vi "VisualizeFlags.vi"() -> ()   [LabVIEW 2017, in "Visualization.lvlib" / "VisualizeFlags.lvclass"]
uses:
  VisualizeFlags.lvclass
  Framework/Bus_class/Bus.lvclass
  VisializeBase_class/Typedefs/VisualizeData.ctl
  VisializeBase_class/Typedefs/clVisualizeData.ctl
  Modules/EventPlugins/EventPluginBaseClass/TypeDefs/clEvtReportArray.ctl
  Modules/EventPlugins/EventPluginBaseClass/TypeDefs/clEvtReport.ctl
  Modules/EventPlugins/EventPluginBaseClass/TypeDefs/dblEvtSignalArray.ctl
  Modules/NetworkImpairmentModule/PublicAPI/Arguments/Broadcasts/dblNetworkTime.ctl
  Modules/NetworkImpairmentModule/PublicAPI/Arguments/Broadcasts/dblPktLoss.ctl
  Modules/FlagImpairModule/PublicAPI/Arguments/Broadcasts/ui32FlagImpairmentArray.ctl
  Framework/Bus_class/Broadcast/Typedefs/clDidInit.ctl
  QMH/Typedefs/clFlagImpairArray.ctl
  VisializeBase_class/Requests/clUserEventType.ctl
  <vilib>/event_ctls.llb/usereventprio.ctl
  <vilib>/Utility/miscctls.llb/LVStringsAndValuesArrayTypeDef_U8.ctl
  QMH/Typedefs/clEvtRptArray.ctl
  QMH/Typedefs/clPmuImpairRptArray.ctl
  QMH/Typedefs/clNetImpairmentTime.ctl
  QMH/Typedefs/clNetIPktLoss.ctl
  QMH/Typedefs/clEvtRptSignal.ctl
  <vilib>/Analysis/baseanly.llb/Mean (DBL).vi
  <vilib>/Waveform/DWDTOps.llb/DWDT Boolean Array to Digital.vi
  <vilib>/Utility/error.llb/Error Cluster From Error Code.vi
  <vilib>/ErrorRing/Error Ring.xnode
  VisializeBase_class/VisualizeBase_class.lvclass
  <userlib>/NIST/NISTErrorLib/NISTErrorLib.lvlib
  Framework/Bus_class/Bus_class.lvlib
  Modules/EventModule/EventModule.lvlib
  Modules/PmuImpairModule/PmuImpairModule.lvlib
  Modules/NetworkImpairmentModule/NetworkImpairmentModule.lvlib
  Modules/FlagImpairModule/FlagImpairModule.lvlib
  Modules/EventPlugins/EventPluginBaseClass/EventPluginBaseClass.lvclass
  <vilib>/Analysis/NI_AALBase.lvlib
  VisualizeApp_class/VisualizeAppBase_class.lvclass
panel:
  out "Error Out":errorcluster[](array[cluster])
  in  "Scrollbar":i32(c297)=20
  in  "QueName":string="FlagQue"
  out "Flags":digitalwaveform(graph)={"t0"=timestamp(0 s since 1904-01-01), "dt"=0.016666666666666666, "Y"={"transitions"=[], "data"=array601x32[19232 elements]}}
  in  "Bus Number":u8(ring) items=["", "1"]
  in  "btnStop":bool
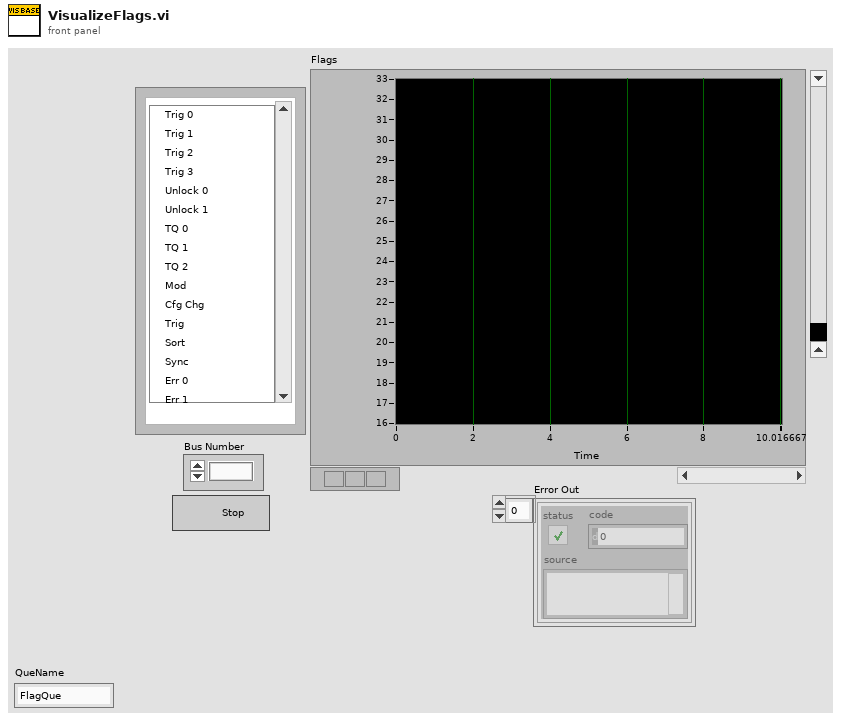
[diagram p1: front panel]
types:
  T1 = typedef "Visualization.lvlib/VisualizeBase_class.lvclass/VisualizeData.ctl" = T2[]
  T2 = typedef "Visualization.lvlib/VisualizeAppBase_class.lvclass/clVisualizeData.ctl" = cluster{"clEvtReportArray":T3, "dblEventSignalArray":T5, "clPmuImpairRptArray":T3, "dblNetworkTime":T6, "dblPktLoss":T7, "FlagImpairArray":T8, "TimeArray":dbl[]}
  T3 = typedef "EventPlugins.lvlib/EventPluginBaseClass.lvclass/clEvtReportArray.ctl" = T4[]
  T4 = typedef "EventPlugins.lvlib/EventPluginBaseClass.lvclass/clEvtReport.ctl" = cluster{"Timestamp":dbl, "Synx":cdb[], "Freq":dbl, "ROCOF":dbl, "ID":i16}
  T5 = typedef "EventPlugins.lvlib/EventPluginBaseClass.lvclass/dblEvtSignalArray.ctl" = dbl[][]
  T6 = typedef "NetworkImpairmentModule.lvlib/dblNetworkTime.ctl" = dbl[]
  T7 = typedef "NetworkImpairmentModule.lvlib/dblPktLoss.ctl" = dbl[]
  T8 = typedef "FlagImpairModule.lvlib/ui32FlagImpairmentArray.ctl" = u32[]
  T9 = typedef "Visualization.lvlib/VisualizeBase_class.lvclass/clRequestEvents.ctl" = cluster{"StopRequest":refnum<user-event>}
  T10 = typedef "Bus_class.lvlib/clBroadcastEvents.ctl" = cluster{"DidInit":refnum<user-event>, "DidStop":refnum<user-event>}
  T11 = typedef "EventModule.lvlib/clBroadcastEvents.ctl" = cluster{"DidInit":refnum<user-event>, "StatusUpdate":refnum<user-event>, "ErrorReport":refnum<user-event>, "DidStop":refnum<user-event>, "ReadEvtConfig":refnum<user-event>, "ReadTimeArray":refnum<user-event>, "ReadEvtParams":refnum<user-event>, "GetEvtReportArray":refnum<user-event>, "ReadPathToPlugin":refnum<user-event>, "GetEvtSignal":refnum<user-event>, "ReadBusNumber":refnum<user-event>}
  T12 = typedef "PmuImpairModule.lvlib/clBroadcastEvents.ctl" = cluster{"DidInit":refnum<user-event>, "StatusUpdate":refnum<user-event>, "ErrorReport":refnum<user-event>, "DidStop":refnum<user-event>, "ImpairConfig":refnum<user-event>, "ImpairParams":refnum<user-event>, "ImpairReports":refnum<user-event>, "PathToPlugin":refnum<user-event>, "BusNumber":refnum<user-event>}
  T13 = typedef "NetworkImpairmentModule.lvlib/clBroadcastEvents.ctl" = cluster{"DidInit":refnum<user-event>, "StatusUpdate":refnum<user-event>, "ErrorReport":refnum<user-event>, "DidStop":refnum<user-event>, "ReadNetImpParams":refnum<user-event>, "ReadLossThreshold":refnum<user-event>, "GetNetworkTime":refnum<user-event>, "GetPktLoss":refnum<user-event>, "ReadPathToPlugin":refnum<user-event>}
  T14 = typedef "FlagImpairModule.lvlib/clBroadcastEvents.ctl" = cluster{"DidInit":refnum<user-event>, "StatusUpdate":refnum<user-event>, "ErrorReport":refnum<user-event>, "DidStop":refnum<user-event>, "ReadFlagImpairConfig":refnum<user-event>, "ReadPluginINIFilePath":refnum<user-event>, "ReadFlagImpairParams":refnum<user-event>, "ReadTimeArray":refnum<user-event>, "GetFlagImpairment":refnum<user-event>}
  T15 = typedef "LVStringsAndValuesArrayTypeDef_U8.ctl" = cluster{"String":string, "Value":u8}[]
  T16 = typedef "Visualization.lvlib/VisualizeBase_class.lvclass/clEvtRptArray.ctl" = cluster{"BusIndex":i32, "clImpairReportArray":T3}
  T17 = typedef "Visualization.lvlib/VisualizeBase_class.lvclass/clPmuImpairRptArray.ctl" = cluster{"BusIndex":i32, "clImpairReportArray":T3}
  T18 = typedef "Visualization.lvlib/VisualizeBase_class.lvclass/clNetImpairmentTime.ctl" = cluster{"BusIndex":i32, "clNetImpairTimeArray":T6}
  T19 = typedef "Visualization.lvlib/VisualizeBase_class.lvclass/clNetIPktLoss.ctl" = cluster{"BusIndex":i32, "clNetPktLoss":T7}
  T20 = typedef "Visualization.lvlib/VisualizeBase_class.lvclass/clFlagImpairArray.ctl" = cluster{"BusIndex":i32, "FlagImpairArray":T8}
  T21 = typedef "Visualization.lvlib/VisualizeBase_class.lvclass/clEvtRptSignal.ctl" = cluster{"BusIndex":i32, "dblEventSignalArray":T5}
  T22 = typedef "Visualization.lvlib/VisualizeBase_class.lvclass/clUserEventType.ctl" = cluster{"BusIndex":i8, "Data":variant}
  T23 = typedef "usereventprio.ctl" = enum32{"high priority", "normal priority"}
  T24 = typedef "Bus_class.lvlib/clDidInit.ctl" = cluster{"Bus":refnum<vi>, "Init?":bool}
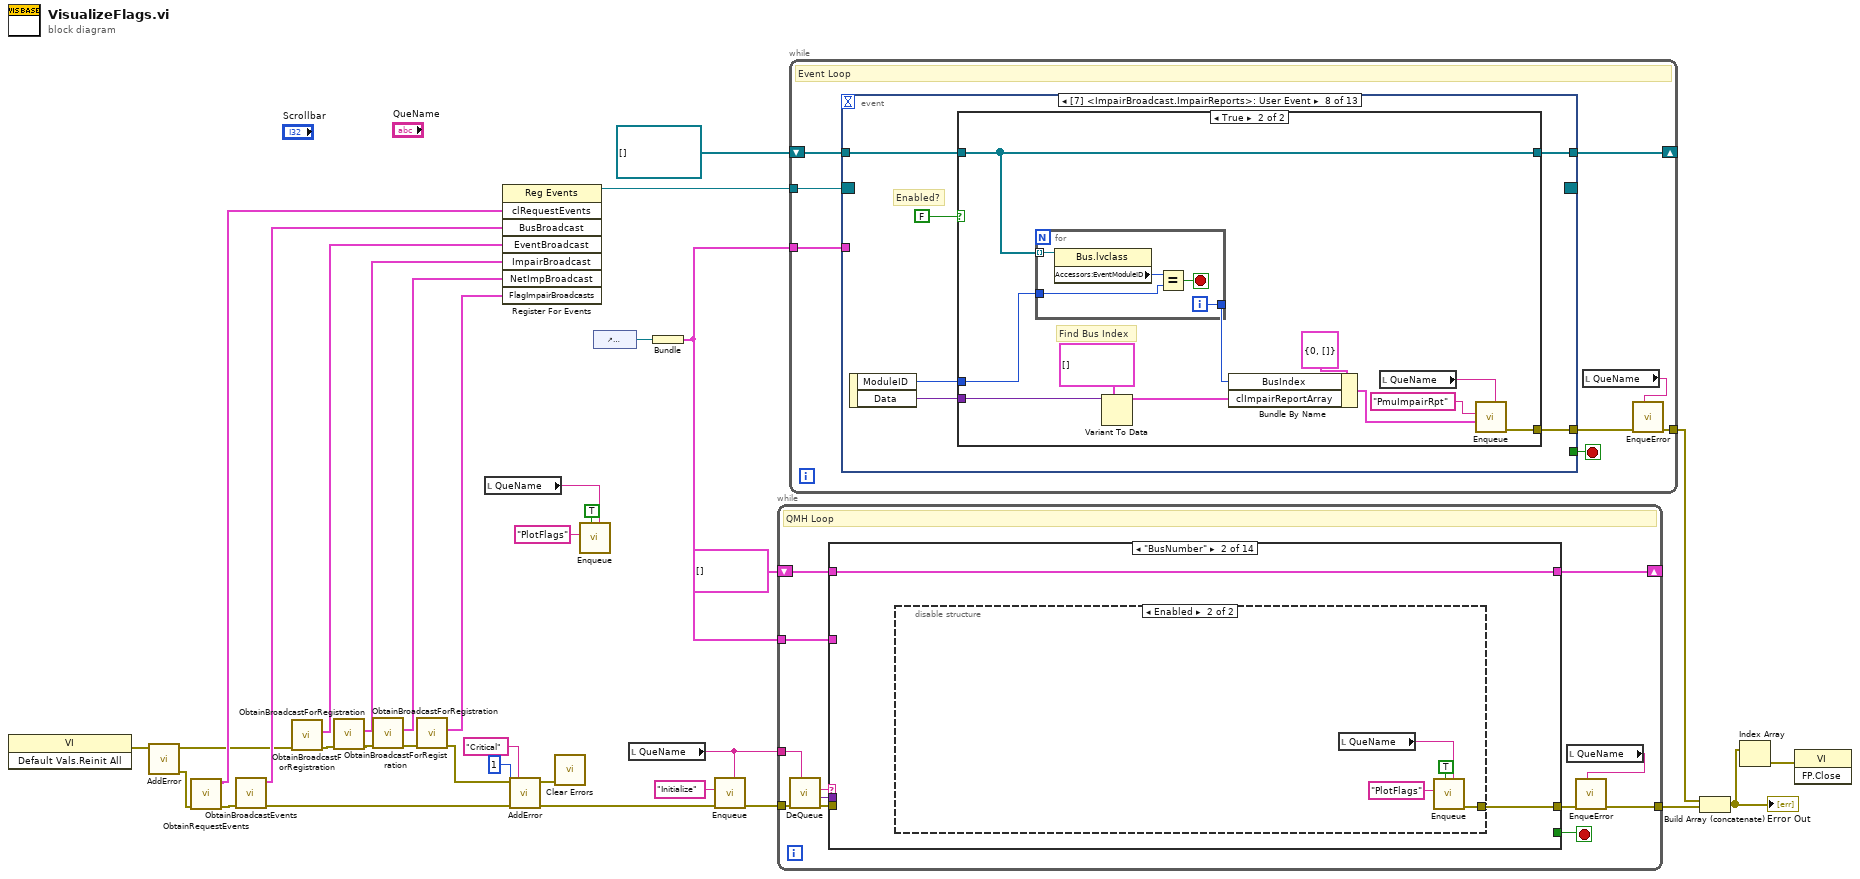
[diagram p0: block diagram]
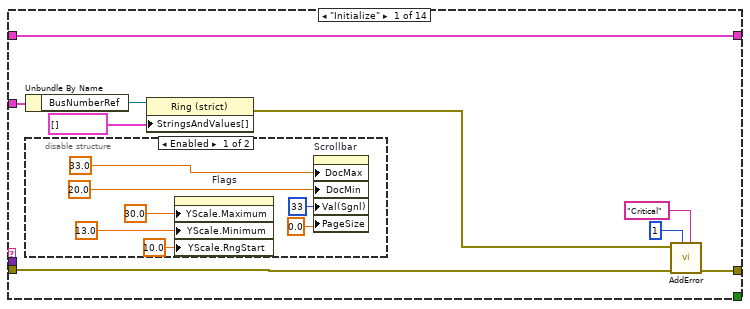
[diagram p2: hidden frame]
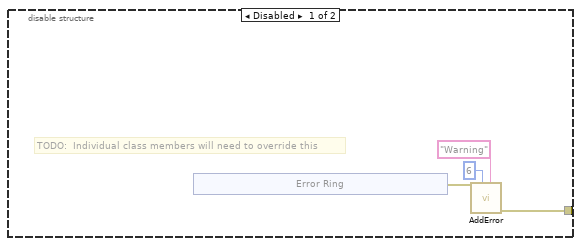
[diagram p4: hidden frame]
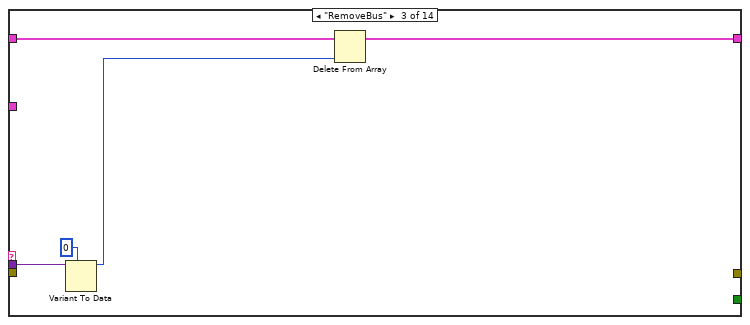
[diagram p5: hidden frame]
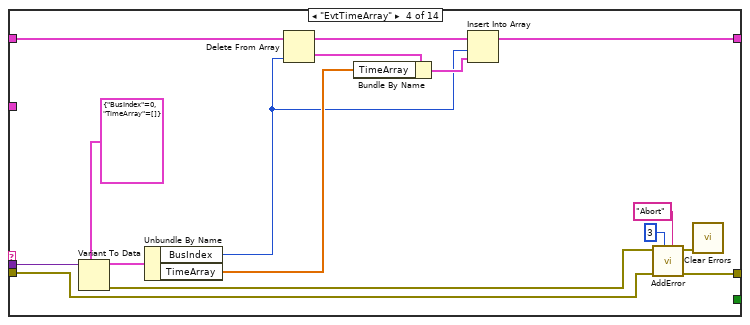
[diagram p6: hidden frame]
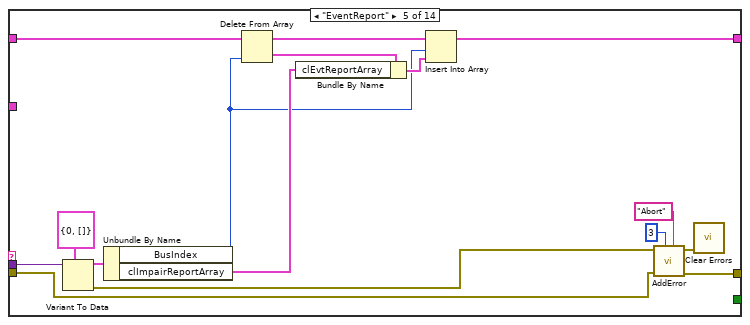
[diagram p7: hidden frame]
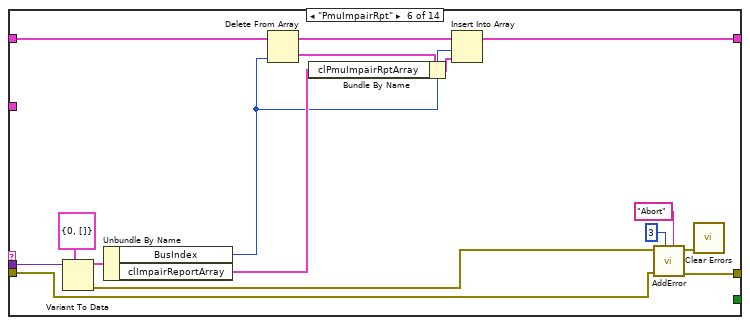
[diagram p8: hidden frame]
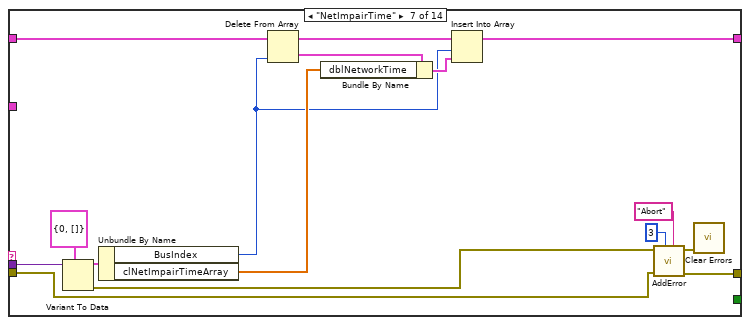
[diagram p9: hidden frame]
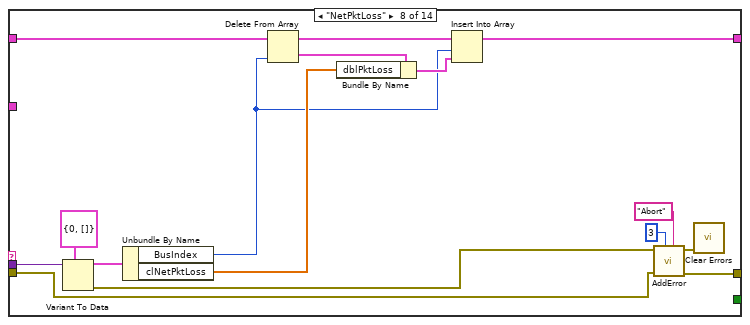
[diagram p10: hidden frame]
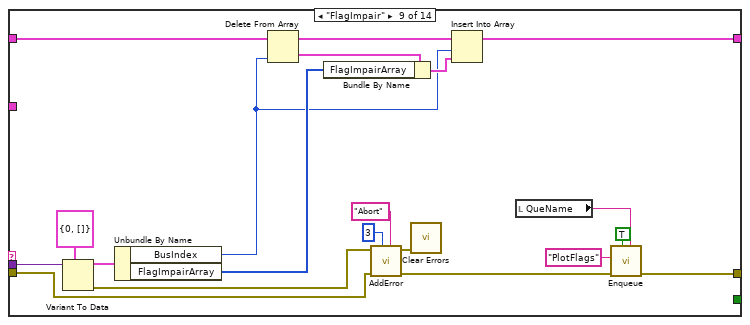
[diagram p11: hidden frame]
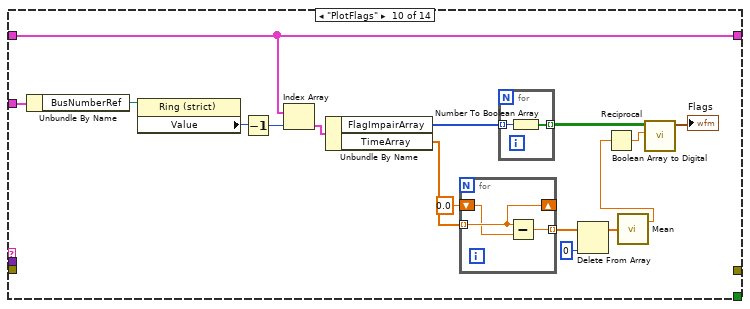
[diagram p12: hidden frame]
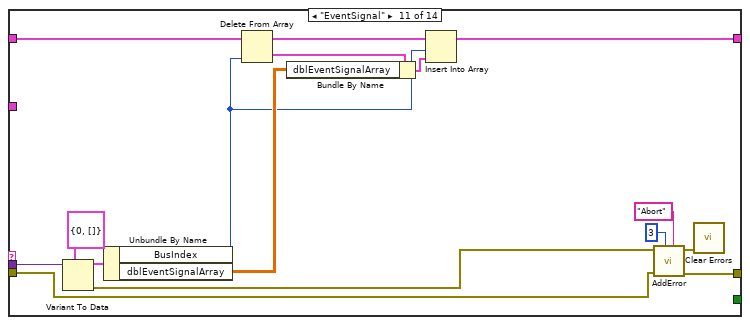
[diagram p13: hidden frame]
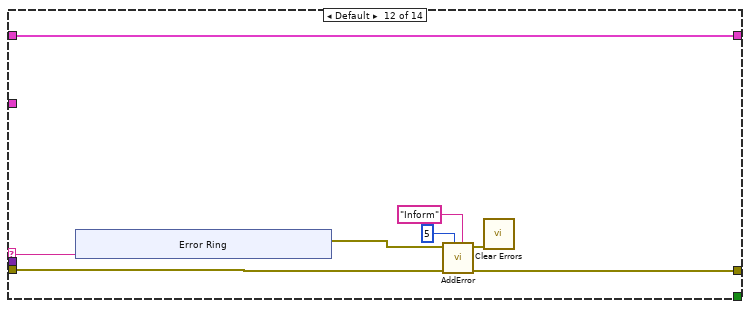
[diagram p14: hidden frame]
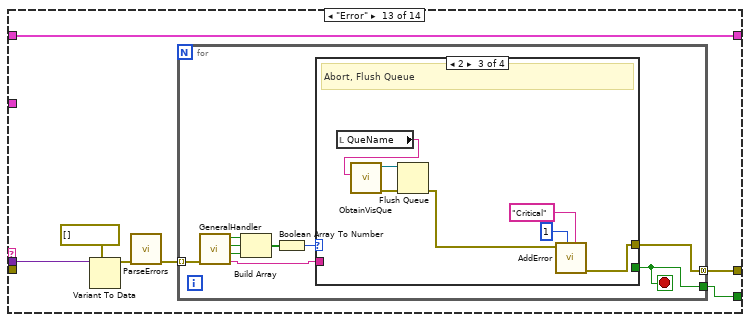
[diagram p15: hidden frame]
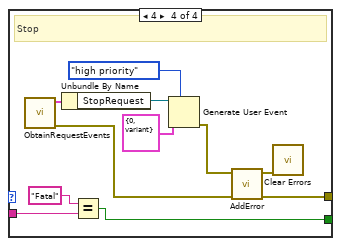
[diagram p18: hidden frame]
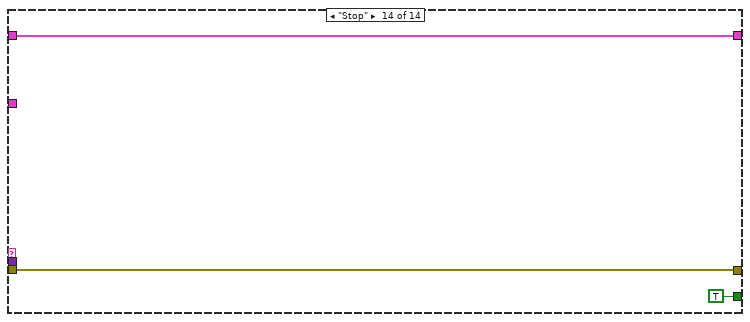
[diagram p19: hidden frame]
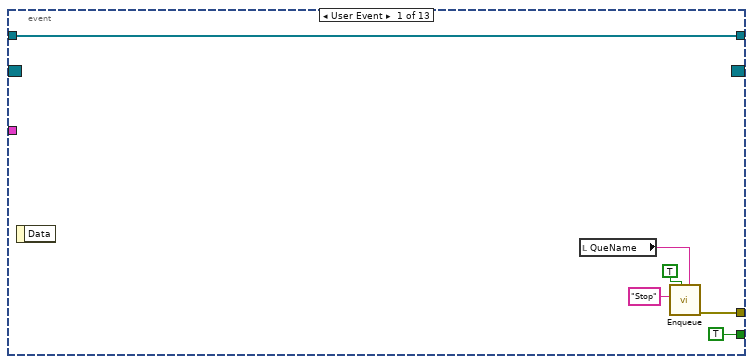
[diagram p20: hidden frame]
diagram:
  n1 = invoke class="VI" method="Default Vals.Reinit All"() -> (error out=w24:errorcluster)  [unwired: 3 in, 2 out]
  n2 = call <userlib>:"AddError.vi"("error in (no error)"=w24) -> ("ErrorArray"=w23:errorcluster[], "error out"=w15:errorcluster)  [unwired: 9 in]
  n3 = call "ObtainRequestEvents.vi"("Error"=w23) -> ("Error"=w28:errorcluster[], "clRequestEvents"=w32:T9)  [unwired: 9 in]
  n4 = call "ObtainBroadcastEvents.vi"("ErrorArray"=w28) -> ("ErrorArray"=w14:errorcluster[], "BusBroadcast"=w27:T10)  [unwired: 9 in]
  n5 = call "ObtainBroadcastForRegistration.vi"("error in (no error)"=w15) -> ("error out"=w18:errorcluster, "EventBroadcast"=w22:T11)  [unwired: 9 in]
  n6 = call "ObtainBroadcastForRegistration.vi"("error in (no error)"=w18) -> ("error out"=w17:errorcluster, "ImpairBroadcast"=w21:T12)  [unwired: 9 in]
  n7 = call "ObtainBroadcastForRegistration.vi"("error in (no error)"=w17) -> ("error out"=w16:errorcluster, "NetImpBroadcast"=w20:T13)  [unwired: 9 in]
  n8 = call "ObtainBroadcastForRegistration.vi"("error in (no error)"=w16) -> ("error out"=w13:errorcluster, "FlagImpairBroadcasts"=w19:T14)  [unwired: 9 in]
  n9 = local read "QueName"() -> (w5:string)
  n10 = register-events(w32, w27, w22, w21, w20, w19) -> (reference out=w31:refnum<event-registration>)  [unwired: 2 in, 1 out]
  n11 = call <userlib>:"AddError.vi"("Severity"="Critical" ("String"), "Priority"=u8 1, "ErrorArray"=w14, "error in (no error)"=w13) -> ("ErrorArray"=w10:errorcluster[], "error out"=w7:errorcluster)  [unwired: 6 in]
  n12 = call <vilib>:"Clear Errors.vi"("error in (no error)"=w7) -> ()  [unwired: 5 in, 2 out]
  n13 = call "Enqueue.vi"("QueName"=w5, "Priority? (F)"=TRUE, "Message"="PlotFlags") -> ()  [unwired: 8 in, 1 out]
  n14 = control-ref of="BusNumberRef"() -> (w26:refnum<vi>)
  n15 = local read "QueName"() -> (w6:string)
  n16 = Bundle("BusNumberRef"=w26) -> (w8:cluster{"BusNumberRef":refnum<vi>})  [unwired: 1 in]
  n17 = call "Enqueue.vi"("QueName"=w6, "Error"=w10, "Message"="Initialize") -> ("Error"=w33:errorcluster[])  [unwired: 8 in]
  n18 = while {
    tunnel: w33 -> [w46]
    tunnel: [w40] -> w30
    tunnel: w8 -> [w39]
    shift-right: [w37] -> _
    shift-left: T1 [] ("VisualizeData") -> [w38]
    tunnel: w6 -> [w36]
    stop <- w41 stop-if-true
    # "QMH Loop"
    n19 = call "DeQueue.vi"("QueName"=w36, "Error"=w46) -> ("Error"=w43:errorcluster[], "Data"=w44:variant, "Message"=w45:string)  [unwired: 7 in]
    n20 = case shown="\"BusNumber\"" w45 {
      selector: w45 -> [_ _ _ _ _ _ _ _ _ _ _ w227 _ _]
      tunnel: w44 -> [_ _ w82 w85 w114 w130 w146 w162 w182 _ w219 _ w241 _]
      tunnel: w43 -> [w52 _ _ w84 w99 w115 w131 w147 w168 _ w204 w225 _ w270]
      tunnel: [w51 w64 _ w83 w104 w120 w136 w152 w166 _ w209 w224 w237 w270] -> w42
      tunnel: [_ _ _ _ _ _ _ _ _ _ _ _ w236 TRUE] -> w41
      tunnel: w39 -> [w55 _ _ _ _ _ _ _ _ w198 _ _ _ _]
      tunnel: w38 -> [w47 w63 w80 w87 w110 w126 w142 w158 w178 w194 w215 w220 w235 w269]
      tunnel: [w47 w63 w79 w86 w111 w127 w143 w159 w179 w194 w216 w220 w235 w269] -> w37
      frame "Initialize" {
        n21 = Unbundle By Name(w55) -> ("BusNumberRef"=w54:refnum<vi>)
        n22 = disable-structure shown="Enabled" {
          frame Enabled {
            n23 = property on="Flags" class="DigitalGraph (strict)"("YScale.Maximum"=30.0 ("Y Scale.Range:Maximum"), "YScale.Minimum"=13.0 ("Y Scale.Range:Maximum"), "YScale.RngStart"=10.0 ("Y Scale.Range:Increment")) -> ()  [unwired: 2 in, 2 out]
            n24 = property on="Scrollbar" class="Scroll (strict)"("DocMax"=33.0 ("Doc Max"), "DocMin"=20.0 ("Doc Min"), "Val(Sgnl)"=33 ("Scrollbar"), "PageSize"=0.0 ("Page Size")) -> ()  [unwired: 2 in, 2 out]
          }
          frame Disabled {
          }
        }
        n25 = property class="Ring (strict)"(reference=w54, "StringsAndValues[]"=T15 [] ("Strings And Values []")) -> (error out=w50:errorcluster)  [unwired: 1 in, 1 out]
        n26 = call <userlib>:"AddError.vi"("Severity"="Critical" ("String"), "Priority"=u8 1, "ErrorArray"=w52, "error in (no error)"=w50) -> ("ErrorArray"=w51:errorcluster[])  [unwired: 6 in, 1 out]
      }
      frame "BusNumber" {
        n27 = disable-structure shown="Enabled" {
          disable-tunnel: [w68 w74] -> w64
          frame Disabled {
            # "TODO:  Individual class members will need to override this"
            n28 = xnode "Error Ring"() -> ("error out"=w67:errorcluster)
            n29 = call <userlib>:"AddError.vi"("Severity"="Warning" ("String"), "Priority"=u8 6, "error in (no error)"=w67) -> ("ErrorArray"=w68:errorcluster[])  [unwired: 7 in, 1 out]
          }
          frame Enabled {
            n30 = local read "QueName"() -> (w75:string)
            n31 = call "Enqueue.vi"("QueName"=w75, "Priority? (F)"=TRUE, "Message"="PlotFlags") -> ("Error"=w74:errorcluster[])  [unwired: 8 in]
          }
        }
      }
      frame "RemoveBus" {
        n32 = Variant To Data(type=0, Variant=w82) -> (data=w78:i32)  [unwired: 1 in, 1 out]
        n33 = Delete From Array(array=w80, index=w78) -> (array with subset deleted=w79:T1)  [unwired: 1 in, 1 out]
      }
      frame "EvtTimeArray" {
        n34 = Variant To Data(type=cluster{"BusIndex":i32, "TimeArray":dbl[]} {"BusIndex"=0, "TimeArray"=[]} ("cluster"), Variant=w85) -> (data=w94:cluster{"BusIndex":i32, "TimeArray":dbl[]}, error out=w98:errorcluster)  [unwired: 1 in]
        n35 = Unbundle By Name(w94) -> ("BusIndex"=w89:i32, "TimeArray"=w91:dbl[])
        n36 = Delete From Array(array=w87, index=w89) -> (deleted portion=w92:T2, array with subset deleted=w93:T1)  [unwired: 1 in]
        n37 = Bundle By Name(cluster=w92, "TimeArray"=w91) -> (w90:T2)
        n38 = Insert Into Array(array=w93, index=w89, new element=w90) -> (w86:T1)
        n39 = call <userlib>:"AddError.vi"("Severity"="Abort" ("String"), "Priority"=u8 3, "ErrorArray"=w84, "error in (no error)"=w98) -> ("ErrorArray"=w83:errorcluster[], "error out"=w97:errorcluster)  [unwired: 6 in]
        n40 = call <vilib>:"Clear Errors.vi"("error in (no error)"=w97) -> ()  [unwired: 5 in, 2 out]
      }
      frame "EventReport" {
        n41 = Variant To Data(type=T16 {"BusIndex"=0, "clImpairReportArray"=[]} ("clEvtReportArray"), Variant=w114) -> (data=w112:T16, error out=w103:errorcluster)  [unwired: 1 in]
        n42 = Unbundle By Name(w112) -> ("BusIndex"=w105:i32, "clImpairReportArray"=w107:T3)
        n43 = Delete From Array(array=w110, index=w105) -> (deleted portion=w108:T2, array with subset deleted=w109:T1)  [unwired: 1 in]
        n44 = Bundle By Name(cluster=w108, "clEvtReportArray"=w107) -> (w106:T2)
        n45 = Insert Into Array(array=w109, index=w105, new element=w106) -> (w111:T1)
        n46 = call <userlib>:"AddError.vi"("Severity"="Abort" ("String"), "Priority"=u8 3, "ErrorArray"=w99, "error in (no error)"=w103) -> ("ErrorArray"=w104:errorcluster[], "error out"=w102:errorcluster)  [unwired: 6 in]
        n47 = call <vilib>:"Clear Errors.vi"("error in (no error)"=w102) -> ()  [unwired: 5 in, 2 out]
      }
      frame "PmuImpairRpt" {
        n48 = Variant To Data(type=T17 {"BusIndex"=0, "clImpairReportArray"=[]} ("clImpairReportArray"), Variant=w130) -> (data=w128:T17, error out=w119:errorcluster)  [unwired: 1 in]
        n49 = Unbundle By Name(w128) -> ("BusIndex"=w121:i32, "clImpairReportArray"=w123:T3)
        n50 = Delete From Array(array=w126, index=w121) -> (deleted portion=w124:T2, array with subset deleted=w125:T1)  [unwired: 1 in]
        n51 = Bundle By Name(cluster=w124, "clPmuImpairRptArray"=w123) -> (w122:T2)
        n52 = Insert Into Array(array=w125, index=w121, new element=w122) -> (w127:T1)
        n53 = call <userlib>:"AddError.vi"("Severity"="Abort" ("String"), "Priority"=u8 3, "ErrorArray"=w115, "error in (no error)"=w119) -> ("ErrorArray"=w120:errorcluster[], "error out"=w118:errorcluster)  [unwired: 6 in]
        n54 = call <vilib>:"Clear Errors.vi"("error in (no error)"=w118) -> ()  [unwired: 5 in, 2 out]
      }
      frame "NetImpairTime" {
        n55 = Variant To Data(type=T18 {"BusIndex"=0, "clNetImpairTimeArray"=[]} ("clImpairReportArray"), Variant=w146) -> (data=w144:T18, error out=w135:errorcluster)  [unwired: 1 in]
        n56 = Unbundle By Name(w144) -> ("BusIndex"=w137:i32, "clNetImpairTimeArray"=w139:T6)
        n57 = Delete From Array(array=w142, index=w137) -> (deleted portion=w140:T2, array with subset deleted=w141:T1)  [unwired: 1 in]
        n58 = Bundle By Name(cluster=w140, "dblNetworkTime"=w139) -> (w138:T2)
        n59 = Insert Into Array(array=w141, index=w137, new element=w138) -> (w143:T1)
        n60 = call <userlib>:"AddError.vi"("Severity"="Abort" ("String"), "Priority"=u8 3, "ErrorArray"=w131, "error in (no error)"=w135) -> ("ErrorArray"=w136:errorcluster[], "error out"=w134:errorcluster)  [unwired: 6 in]
        n61 = call <vilib>:"Clear Errors.vi"("error in (no error)"=w134) -> ()  [unwired: 5 in, 2 out]
      }
      frame "NetPktLoss" {
        n62 = Variant To Data(type=T19 {"BusIndex"=0, "clNetPktLoss"=[]} ("clNetPktLoss"), Variant=w162) -> (data=w160:T19, error out=w151:errorcluster)  [unwired: 1 in]
        n63 = Unbundle By Name(w160) -> ("BusIndex"=w153:i32, "clNetPktLoss"=w155:T7)
        n64 = Delete From Array(array=w158, index=w153) -> (deleted portion=w156:T2, array with subset deleted=w157:T1)  [unwired: 1 in]
        n65 = Bundle By Name(cluster=w156, "dblPktLoss"=w155) -> (w154:T2)
        n66 = Insert Into Array(array=w157, index=w153, new element=w154) -> (w159:T1)
        n67 = call <userlib>:"AddError.vi"("Severity"="Abort" ("String"), "Priority"=u8 3, "ErrorArray"=w147, "error in (no error)"=w151) -> ("ErrorArray"=w152:errorcluster[], "error out"=w150:errorcluster)  [unwired: 6 in]
        n68 = call <vilib>:"Clear Errors.vi"("error in (no error)"=w150) -> ()  [unwired: 5 in, 2 out]
      }
      frame "FlagImpair" {
        n69 = Variant To Data(type=T20 {"BusIndex"=0, "FlagImpairArray"=[]} ("clFlagImpairArray"), Variant=w182) -> (data=w180:T20, error out=w172:errorcluster)  [unwired: 1 in]
        n70 = Unbundle By Name(w180) -> ("BusIndex"=w173:i32, "FlagImpairArray"=w175:T8)
        n71 = Delete From Array(array=w178, index=w173) -> (deleted portion=w176:T2, array with subset deleted=w177:T1)  [unwired: 1 in]
        n72 = Bundle By Name(cluster=w176, "FlagImpairArray"=w175) -> (w174:T2)
        n73 = call <userlib>:"AddError.vi"("Severity"="Abort" ("String"), "Priority"=u8 3, "ErrorArray"=w168, "error in (no error)"=w172) -> ("ErrorArray"=w167:errorcluster[], "error out"=w171:errorcluster)  [unwired: 6 in]
        n74 = call <vilib>:"Clear Errors.vi"("error in (no error)"=w171) -> ()  [unwired: 5 in, 2 out]
        n75 = Insert Into Array(array=w177, index=w173, new element=w174) -> (w179:T1)
        n76 = local read "QueName"() -> (w163:string)
        n77 = call "Enqueue.vi"("QueName"=w163, "Priority? (F)"=TRUE, "Error"=w167, "Message"="PlotFlags") -> ("Error"=w166:errorcluster[])  [unwired: 7 in]
      }
      frame "PlotFlags" {
        n78 = Unbundle By Name(w198) -> ("BusNumberRef"=w197:refnum<vi>)
        n79 = property class="Ring (strict)"(reference=w197) -> ("Value"=w196:u8)  [unwired: 1 in, 2 out]
        n80 = Decrement(x=w196) -> (x-1=w195:u8)
        n81 = Index Array(array=w194, index=w195) -> (element=w193:T2)
        n82 = Unbundle By Name(w193) -> ("FlagImpairArray"=w192:T8, "TimeArray"=w190:dbl[])
        n83 = for {
          tunnel: w190 -> [w200] mode=indexing
          shift-right: [w200] -> _
          shift-left: 0.0 ("Numeric") -> [w199]
          tunnel: [w201] -> w188 mode=indexing
          n84 = Subtract(x=w200, y=w199) -> (x-y=w201:dbl)
        }
        n85 = for {
          tunnel: w192 -> [w203] mode=indexing
          tunnel: [w202] -> w191 mode=indexing
          n86 = Number To Boolean Array(number=w203) -> (Boolean array=w202:bool[])
        }
        n87 = Delete From Array(array=w188, index=0) -> (array with subset deleted=w186:dbl[])  [unwired: 1 in, 1 out]
        n88 = call-poly <vilib>:"Mean.vi"("X"=w186) -> ("mean"=w185:dbl)  [unwired: 1 out]
        n89 = Reciprocal(x=w185) -> (1/x=w183:dbl)
        n90 = call-poly <vilib>:"Boolean Array to Digital.vi"("sample rate"=w183, "boolean array"=w191) -> ("digital waveform"=→"Flags":digitalwaveform)  [unwired: 8 in, 1 out]
      }
      frame "EventSignal" {
        n91 = Variant To Data(type=T21 {"BusIndex"=0, "dblEventSignalArray"=[]} ("clEvtReportArray"), Variant=w219) -> (data=w217:T21, error out=w208:errorcluster)  [unwired: 1 in]
        n92 = Unbundle By Name(w217) -> ("BusIndex"=w210:i32, "dblEventSignalArray"=w212:T5)
        n93 = Delete From Array(array=w215, index=w210) -> (deleted portion=w213:T2, array with subset deleted=w214:T1)  [unwired: 1 in]
        n94 = Bundle By Name(cluster=w213, "dblEventSignalArray"=w212) -> (w211:T2)
        n95 = Insert Into Array(array=w214, index=w210, new element=w211) -> (w216:T1)
        n96 = call <userlib>:"AddError.vi"("Severity"="Abort" ("String"), "Priority"=u8 3, "ErrorArray"=w204, "error in (no error)"=w208) -> ("ErrorArray"=w209:errorcluster[], "error out"=w207:errorcluster)  [unwired: 6 in]
        n97 = call <vilib>:"Clear Errors.vi"("error in (no error)"=w207) -> ()  [unwired: 5 in, 2 out]
      }
      frame Default {
        n98 = xnode "Error Ring"("parameter 0"=w227) -> ("error out"=w226:errorcluster)
        n99 = call <userlib>:"AddError.vi"("Severity"="Inform" ("String"), "Priority"=u8 5, "ErrorArray"=w225, "error in (no error)"=w226) -> ("ErrorArray"=w224:errorcluster[], "error out"=w223:errorcluster)  [unwired: 6 in]
        n100 = call <vilib>:"Clear Errors.vi"("error in (no error)"=w223) -> ()  [unwired: 5 in, 2 out]
      }
      frame "Error" {
        n101 = Variant To Data(type=errorcluster[] [], Variant=w241) -> (data=w239:errorcluster[])  [unwired: 1 in, 1 out]
        n102 = call <userlib>:"ParseErrors.vi"("ErrorArray"=w239) -> ("ErrorArray"=w238:errorcluster[])  [unwired: 8 in, 2 out]
        n103 = for {
          tunnel: w238 -> [w250] mode=indexing
          tunnel: [w244] -> w237 mode=concatenating
          tunnel: [w242] -> w236
          stop <- w242 stop-if-true
          n104 = call <userlib>:"GeneralHandler.vi"("error in (no error)"=w250) -> ("Severity"=w243:string, "Stop"=w247:bool, "Abort"=w248:bool, "Continue"=w249:bool)  [unwired: 7 in]
          n105 = Build Array(w249, w248, w247) -> (w246:bool[])
          n106 = Boolean Array To Number(Boolean array=w246) -> (number=w245:u32)
          n107 = case shown="2" w245 {
            tunnel: [_ _ w255 w266] -> w244
            tunnel: w243 -> [_ _ _ w260]
            tunnel: [_ _ _ w258] -> w242
            frame 0, Default {
              # "No Dialog"
            }
            frame 1 {
              # "Continue"
            }
            frame 2 {
              # "Abort, Flush Queue"
              n108 = local read "QueName"() -> (w251:string)
              n109 = call "ObtainVisQue.vi"("QueName"=w251) -> ("error out"=w257:errorcluster, "queue out"=w256:refnum<queue>)  [unwired: 9 in]
              n110 = Flush Queue(queue=w256, error in (no error)=w257) -> (error out=w254:errorcluster)  [unwired: 2 out]
              n111 = call <userlib>:"AddError.vi"("Severity"="Critical" ("String"), "Priority"=u8 1, "error in (no error)"=w254) -> ("ErrorArray"=w255:errorcluster[])  [unwired: 7 in, 1 out]
            }
            frame 4 {
              # "Stop"
              n112 = call "ObtainRequestEvents.vi"() -> ("Error"=w264:errorcluster[], "clRequestEvents"=w268:T9)  [unwired: 10 in]
              n113 = Unbundle By Name(w268) -> ("StopRequest"=w267:refnum<user-event>)
              n114 = Equal?(x="Fatal", y=w260) -> (x = y?=w258:bool)
              n115 = Generate User Event(priority (normal)=usereventprio."high priority", user event=w267, event data cluster=T22 {"BusIndex"=0, "Data"=variant} ("event data")) -> (error out=w265:errorcluster)  [unwired: 1 in, 1 out]
              n116 = call <userlib>:"AddError.vi"("ErrorArray"=w264, "error in (no error)"=w265) -> ("ErrorArray"=w266:errorcluster[], "error out"=w261:errorcluster)  [unwired: 8 in]
              n117 = call <vilib>:"Clear Errors.vi"("error in (no error)"=w261) -> ()  [unwired: 5 in, 2 out]
            }
          }
        }
      }
      frame "Stop" {
      }
    }
    n118 = local read "QueName"() -> (w35:string)
    n119 = call "EnqueError.vi"("QueName"=w35, "Error"=w42) -> ("Error"=w40:errorcluster[])  [unwired: 9 in]
  }
  n120 = while {
    tunnel: w31 -> [w279]
    tunnel: [w276] -> w29
    tunnel: w8 -> [w275]
    shift-right: [w273] -> _
    shift-left: refnum<class "Bus.lvclass">[] [] -> [w274]
    stop <- w278 stop-if-true
    # "Event Loop"
    n121 = event shown="[7] <ImpairBroadcast.ImpairReports>: User Event" {
      selector: w279 -> [_ _ _ _ _ _ _ _ _ _ _ _ _]
      dyn-events: [_ _ w299 _ _ _ _ _ _ _ _ _ _] -> _
      timeout: _ -> [_ _ _ _ _ _ _ _ _ _ _ _ _]
      tunnel: [TRUE _ _ _ _ _ _ _ _ _ _ _ _] -> w278
      tunnel: [w284 w290 w302 w320 w327 w353 w378 w401 w424 w447 w470 _ w503] -> w277
      tunnel: w275 -> [_ _ w312 w324 _ _ _ _ _ _ _ _ _]
      tunnel: w274 -> [w281 w287 w311 w323 w330 w351 w381 w404 w427 w450 w473 w491 w497]
      tunnel: [w281 w287 w308 w322 w325 w352 w376 w399 w422 w445 w468 w491 w497] -> w273
      event User Event {
        n122 = event-data() -> ()  [unwired: 1 in, 1 out]
        n123 = local read "QueName"() -> (w280:string)
        n124 = call "Enqueue.vi"("QueName"=w280, "Priority? (F)"=TRUE, "Message"="Stop") -> ("Error"=w284:errorcluster[])  [unwired: 8 in]
      }
      event "Bus Number": Value Change {
        n125 = event-data() -> ("NewVal"=w289:u8)  [unwired: 1 in]
        n126 = local read "QueName"() -> (w286:string)
        n127 = call "Enqueue.vi"("QueName"=w286, "Data"=w289, "Message"="BusNumber") -> ("Error"=w290:errorcluster[])  [unwired: 8 in]
      }
      event User Event {
        n128 = event-data() -> ("Data"=w315:variant)  [unwired: 1 in]
        n129 = Unbundle By Name(w312) -> ("BusNumberRef"=w310:refnum<vi>)
        n130 = Variant To Data(type=T24 {"Bus"=refnum, "Init?"=FALSE} ("clBusDidInit"), Variant=w315) -> (data=w313:T24)  [unwired: 1 in, 1 out]
        n131 = Unbundle By Name(w313) -> ("Bus"=w309:refnum<vi>)
        n132 = call "AddBus.vi"("BusRef"=w309, "BusNumberRef"=w310, "BusArray"=w311) -> ("BusArray"=w308:refnum<class "Bus.lvclass">[])  [unwired: 8 in]
        n133 = call "ObtainRequestEvents.vi"() -> ("Error"=w294:errorcluster[], "clRequestEvents"=w292:T9)  [unwired: 10 in]
        n134 = call "ObtainBroadcastEvents.vi"("ErrorArray"=w294) -> ("ErrorArray"=w293:errorcluster[], "BusBroadcast"=w291:T10)  [unwired: 9 in]
        n135 = call "ObtainBroadcastForRegistration.vi"() -> ("error out"=w307:errorcluster, "EventBroadcast"=w298:T11)  [unwired: 10 in]
        n136 = call "ObtainBroadcastForRegistration.vi"("error in (no error)"=w307) -> ("error out"=w306:errorcluster, "ImpairBroadcast"=w297:T12)  [unwired: 9 in]
        n137 = call "ObtainBroadcastForRegistration.vi"("error in (no error)"=w306) -> ("error out"=w305:errorcluster, "NetImpBroadcast"=w296:T13)  [unwired: 9 in]
        n138 = call "ObtainBroadcastForRegistration.vi"("error in (no error)"=w305) -> ("error out"=w300:errorcluster, "FlagImpairBroadcasts"=w295:T14)  [unwired: 9 in]
        n139 = register-events(w292, w291, w298, w297, w296, w295) -> (reference out=w299:refnum<event-registration>)  [unwired: 2 in, 1 out]
        n140 = call <userlib>:"AddError.vi"("Severity"="Critical" ("String"), "Priority"=u8 1, "ErrorArray"=w293, "error in (no error)"=w300) -> ("ErrorArray"=w302:errorcluster[], "error out"=w301:errorcluster)  [unwired: 6 in]
        n141 = call <vilib>:"Clear Errors.vi"("error in (no error)"=w301) -> ()  [unwired: 5 in, 2 out]
      }
      event User Event {
        n142 = event-data() -> ("BusNumber"=w317:i8)  [unwired: 1 in]
        n143 = Unbundle By Name(w324) -> ("BusNumberRef"=w321:refnum<vi>)
        n144 = call "RemoveBus.vi"("BusArray"=w323, "BusNumberRef"=w321, "BusNumber"=w317) -> ("BusArray"=w322:refnum<class "Bus.lvclass">[], "BusIndex"=w319:i32)  [unwired: 6 in]
        n145 = local read "QueName"() -> (w316:string)
        n146 = call "Enqueue.vi"("QueName"=w316, "Data"=w319, "Message"="RemoveBus") -> ("Error"=w320:errorcluster[])  [unwired: 8 in]
      }
      event User Event {
        # "Enabled?"
        n147 = event-data() -> ("ModuleID"=w329:i32, "Data"=w328:variant)  [unwired: 1 in]
        n148 = case shown="False" FALSE {
          tunnel: w330 -> [w331 w333]
          tunnel: w329 -> [_ w342]
          tunnel: w328 -> [_ w340]
          tunnel: [_ w337] -> w327
          tunnel: [w331 w333] -> w325
          frame False {
          }
          frame True {
            # "Find Bus Index"
            n149 = for {
              tunnel: w333 -> [w347] mode=indexing
              tunnel: w342 -> [w345]
              tunnel: [w343] -> w341
              i -> [w343]
              stop <- w344 stop-if-true
              n150 = property class="Bus.lvclass"(reference=w347) -> ("Accessors:EventModuleID"=w346:i32)  [unwired: 1 in, 2 out]
              n151 = Equal?(x=w346, y=w345) -> (x = y?=w344:bool)
            }
            n152 = Variant To Data(type=T3 [] ("clEvtReportArray"), Variant=w340) -> (data=w338:T3)  [unwired: 1 in, 1 out]
            n153 = Bundle By Name(cluster=T16 {"BusIndex"=0, "clImpairReportArray"=[]} ("clEvtReportArray"), "BusIndex"=w341, "clImpairReportArray"=w338) -> (w336:T16)
            n154 = local read "QueName"() -> (w332:string)
            n155 = call "Enqueue.vi"("QueName"=w332, "Data"=w336, "Message"="EventReport") -> ("Error"=w337:errorcluster[])  [unwired: 8 in]
          }
        }
      }
      event User Event {
        w348 = TRUE  # Enabled?
        n156 = event-data() -> ("ModuleID"=w350:i32, "Data"=w349:variant)  [unwired: 1 in]
        n157 = case shown="True" w348 {
          tunnel: [w354 w370] -> w352
          tunnel: w351 -> [w354 w370]
          tunnel: w350 -> [_ w367]
          tunnel: w349 -> [_ w369]
          tunnel: [_ w357] -> w353
          frame False {
          }
          frame True {
            n158 = Variant To Data(type=dbl[] [], Variant=w369) -> (data=w366:dbl[], error out=w362:errorcluster)  [unwired: 1 in]
            n159 = for {
              tunnel: w370 -> [w375] mode=indexing
              tunnel: w367 -> [w373]
              tunnel: [w371] -> w356
              i -> [w371]
              stop <- w372 stop-if-true
              # "Find Bus Index"
              n160 = property class="Bus.lvclass"(reference=w375) -> ("Accessors:EventModuleID"=w374:i32)  [unwired: 1 in, 2 out]
              n161 = Equal?(x=w374, y=w373) -> (x = y?=w372:bool)
            }
            n162 = call <userlib>:"AddError.vi"("Severity"="Critical" ("String"), "Priority"=u8 1, "error in (no error)"=w362) -> ("ErrorArray"=w358:errorcluster[], "error out"=w361:errorcluster)  [unwired: 7 in]
            n163 = call <vilib>:"Clear Errors.vi"("error in (no error)"=w361) -> ()  [unwired: 5 in, 2 out]
            n164 = Bundle(w356, w366) -> (w365:cluster{i32, dbl[]})  [unwired: 1 in]
            n165 = To Variant(anything=w365) -> (Variant=w364:variant)
            n166 = local read "QueName"() -> (w355:string)
            n167 = call "Enqueue.vi"("QueName"=w355, "Error"=w358, "Data"=w364, "Message"="EvtTimeArray") -> ("Error"=w357:errorcluster[])  [unwired: 7 in]
          }
        }
      }
      event User Event {
        # "Enabled?"
        n168 = event-data() -> ("ModuleID"=w380:i32, "Data"=w379:variant)  [unwired: 1 in]
        n169 = case shown="False" FALSE {
          tunnel: w381 -> [w382 w384]
          tunnel: w380 -> [_ w393]
          tunnel: w379 -> [_ w391]
          tunnel: [_ w388] -> w378
          tunnel: [w382 w384] -> w376
          frame False {
          }
          frame True {
            # "Find Bus Index"
            n170 = for {
              tunnel: w384 -> [w398] mode=indexing
              tunnel: w393 -> [w396]
              tunnel: [w394] -> w392
              i -> [w394]
              stop <- w395 stop-if-true
              n171 = property class="Bus.lvclass"(reference=w398) -> ("Accessors:EventModuleID"=w397:i32)  [unwired: 1 in, 2 out]
              n172 = Equal?(x=w397, y=w396) -> (x = y?=w395:bool)
            }
            n173 = Variant To Data(type=T5 [] ("dblEventSignalArray"), Variant=w391) -> (data=w389:T5)  [unwired: 1 in, 1 out]
            n174 = Bundle By Name(cluster=T21 {"BusIndex"=0, "dblEventSignalArray"=[]} ("clEvtReportArray"), "BusIndex"=w392, "dblEventSignalArray"=w389) -> (w387:T21)
            n175 = local read "QueName"() -> (w383:string)
            n176 = call "Enqueue.vi"("QueName"=w383, "Data"=w387, "Message"="EventSignal") -> ("Error"=w388:errorcluster[])  [unwired: 8 in]
          }
        }
      }
      event User Event {
        # "Enabled?"
        n177 = event-data() -> ("ModuleID"=w403:i32, "Data"=w402:variant)  [unwired: 1 in]
        n178 = case shown="True" FALSE {
          tunnel: w404 -> [w405 w407]
          tunnel: w403 -> [_ w416]
          tunnel: w402 -> [_ w414]
          tunnel: [_ w411] -> w401
          tunnel: [w405 w407] -> w399
          frame False {
          }
          frame True {
            # "Find Bus Index"
            n179 = for {
              tunnel: w407 -> [w421] mode=indexing
              tunnel: w416 -> [w419]
              tunnel: [w417] -> w415
              i -> [w417]
              stop <- w418 stop-if-true
              n180 = property class="Bus.lvclass"(reference=w421) -> ("Accessors:EventModuleID"=w420:i32)  [unwired: 1 in, 2 out]
              n181 = Equal?(x=w420, y=w419) -> (x = y?=w418:bool)
            }
            n182 = Variant To Data(type=T3 [] ("clEvtReportArray"), Variant=w414) -> (data=w412:T3)  [unwired: 1 in, 1 out]
            n183 = Bundle By Name(cluster=T17 {"BusIndex"=0, "clImpairReportArray"=[]} ("clEvtReportArray"), "BusIndex"=w415, "clImpairReportArray"=w412) -> (w410:T17)
            n184 = local read "QueName"() -> (w406:string)
            n185 = call "Enqueue.vi"("QueName"=w406, "Data"=w410, "Message"="PmuImpairRpt") -> ("Error"=w411:errorcluster[])  [unwired: 8 in]
          }
        }
      }
      event User Event {
        # "Enabled?"
        n186 = event-data() -> ("ModuleID"=w426:i32, "Data"=w425:variant)  [unwired: 1 in]
        n187 = case shown="False" FALSE {
          tunnel: w427 -> [w428 w430]
          tunnel: w426 -> [_ w439]
          tunnel: w425 -> [_ w437]
          tunnel: [_ w434] -> w424
          tunnel: [w428 w430] -> w422
          frame False {
          }
          frame True {
            # "Find Bus Index"
            n188 = for {
              tunnel: w430 -> [w444] mode=indexing
              tunnel: w439 -> [w442]
              tunnel: [w440] -> w438
              i -> [w440]
              stop <- w441 stop-if-true
              n189 = property class="Bus.lvclass"(reference=w444) -> ("Accessors:EventModuleID"=w443:i32)  [unwired: 1 in, 2 out]
              n190 = Equal?(x=w443, y=w442) -> (x = y?=w441:bool)
            }
            n191 = Variant To Data(type=T6 [] ("dblNetworkTime"), Variant=w437) -> (data=w435:T6)  [unwired: 1 in, 1 out]
            n192 = Bundle By Name(cluster=T18 {"BusIndex"=0, "clNetImpairTimeArray"=[]} ("clEvtReportArray"), "BusIndex"=w438, "clNetImpairTimeArray"=w435) -> (w433:T18)
            n193 = local read "QueName"() -> (w429:string)
            n194 = call "Enqueue.vi"("QueName"=w429, "Data"=w433, "Message"="NetImpairTime") -> ("Error"=w434:errorcluster[])  [unwired: 8 in]
          }
        }
      }
      event User Event {
        # "Enabled?"
        n195 = event-data() -> ("ModuleID"=w449:i32, "Data"=w448:variant)  [unwired: 1 in]
        n196 = case shown="False" FALSE {
          tunnel: w450 -> [w451 w453]
          tunnel: w449 -> [_ w462]
          tunnel: w448 -> [_ w460]
          tunnel: [_ w457] -> w447
          tunnel: [w451 w453] -> w445
          frame False {
          }
          frame True {
            # "Find Bus Index"
            n197 = for {
              tunnel: w453 -> [w467] mode=indexing
              tunnel: w462 -> [w465]
              tunnel: [w463] -> w461
              i -> [w463]
              stop <- w464 stop-if-true
              n198 = property class="Bus.lvclass"(reference=w467) -> ("Accessors:EventModuleID"=w466:i32)  [unwired: 1 in, 2 out]
              n199 = Equal?(x=w466, y=w465) -> (x = y?=w464:bool)
            }
            n200 = Variant To Data(type=T7 [] ("dblPktLoss"), Variant=w460) -> (data=w458:T7)  [unwired: 1 in, 1 out]
            n201 = Bundle By Name(cluster=T19 {"BusIndex"=0, "clNetPktLoss"=[]} ("clEvtReportArray"), "BusIndex"=w461, "clNetPktLoss"=w458) -> (w456:T19)
            n202 = local read "QueName"() -> (w452:string)
            n203 = call "Enqueue.vi"("QueName"=w452, "Data"=w456, "Message"="NetPktLoss") -> ("Error"=w457:errorcluster[])  [unwired: 8 in]
          }
        }
      }
      event User Event {
        # "Enabled?"
        n204 = event-data() -> ("ModuleID"=w472:i32, "Data"=w471:variant)  [unwired: 1 in]
        n205 = case shown="True" TRUE {
          tunnel: w473 -> [w474 w476]
          tunnel: w472 -> [_ w485]
          tunnel: w471 -> [_ w483]
          tunnel: [_ w480] -> w470
          tunnel: [w474 w476] -> w468
          frame False {
          }
          frame True {
            # "Find Bus Index"
            n206 = for {
              tunnel: w476 -> [w490] mode=indexing
              tunnel: w485 -> [w488]
              tunnel: [w486] -> w484
              i -> [w486]
              stop <- w487 stop-if-true
              n207 = property class="Bus.lvclass"(reference=w490) -> ("Accessors:EventModuleID"=w489:i32)  [unwired: 1 in, 2 out]
              n208 = Equal?(x=w489, y=w488) -> (x = y?=w487:bool)
            }
            n209 = Variant To Data(type=T8 [] ("ui32FlagImpairmentArray"), Variant=w483) -> (data=w481:T8)  [unwired: 1 in, 1 out]
            n210 = Bundle By Name(cluster=T20 {"BusIndex"=0, "FlagImpairArray"=[]} ("clEvtReportArray"), "BusIndex"=w484, "FlagImpairArray"=w481) -> (w479:T20)
            n211 = local read "QueName"() -> (w475:string)
            n212 = call "Enqueue.vi"("QueName"=w475, "Data"=w479, "Message"="FlagImpair") -> ("Error"=w480:errorcluster[])  [unwired: 8 in]
          }
        }
      }
      event "Scrollbar": Value Change {
        n213 = event-data() -> ("NewVal"=w492:i32)  [unwired: 1 in]
        n214 = property on="Flags" class="DigitalGraph (strict)"() -> ("YScale.Maximum"=w496:dbl, "YScale.Minimum"=w495:dbl)  [unwired: 2 in, 2 out]
        n215 = Subtract(x=w496, y=w495) -> (x-y=w494:dbl)
        n216 = Subtract(x=w492, y=w494) -> (x-y=w493:dbl)
        n217 = property on="Flags" class="DigitalGraph (strict)"("YScale.Maximum"=w492, "YScale.Minimum"=w493) -> ()  [unwired: 2 in, 2 out]
      }
      event "btnStop": Value Change {
        n218 = event-data() -> ()  [unwired: 1 in, 1 out]
        n219 = call "ObtainRequestEvents.vi"() -> ("Error"=w507:errorcluster[], "clRequestEvents"=w504:T9)  [unwired: 10 in]
        n220 = Unbundle By Name(w504) -> ("StopRequest"=w505:refnum<user-event>)
        n221 = Generate User Event(priority (normal)=usereventprio."high priority", user event=w505, event data cluster=T22 {"BusIndex"=0, "Data"=variant} ("event data")) -> (error out=w506:errorcluster)  [unwired: 1 in, 1 out]
        n222 = call <userlib>:"AddError.vi"("Severity"="Fatal" ("String"), "Priority"=u8 0, "ErrorArray"=w507, "error in (no error)"=w506) -> ("ErrorArray"=w503:errorcluster[], "error out"=w500:errorcluster)  [unwired: 6 in]
        n223 = call <vilib>:"Clear Errors.vi"("error in (no error)"=w500) -> ()  [unwired: 5 in, 2 out]
      }
    }
    n224 = local read "QueName"() -> (w272:string)
    n225 = call "EnqueError.vi"("QueName"=w272, "Error"=w277) -> ("Error"=w276:errorcluster[])  [unwired: 9 in]
  }
  n226 = Build Array (concatenate)(w29, w30) -> (w2:errorcluster[])
  "Error Out" <- w2
  n227 = Index Array(array=w2) -> (element=w1:errorcluster)  [unwired: 1 in]
  n228 = invoke class="VI" method="FP.Close"(error in=w1) -> ()  [unwired: 2 in, 3 out]
